vi "FPGA Main.vi"() -> ()   [LabVIEW 2016]
uses:
  Program Files (x86)/National Instruments/LabVIEW 2016/examples/roboRIO/Customized FPGA/Sub VIs/Utilities/Start Boolean.ctl
  <vilib>/Platform/TimedLoop/XDataNode/timing_clust.ctl
  <vilib>/Platform/TimedLoop/XDataNode/nitl_modes.ctl
  <vilib>/Platform/TimedLoop/XDataNode/wakeup.ctl
  <vilib>/rvi/Emulation/niFpgaGetClockAttributes.vi
  <vilib>/rvi/Emulation/niFpgaSctlEmulationGetInTimedLoop.vi
  <vilib>/rvi/Emulation/niFpgaEmulationReportErrorSimple.vi
  <vilib>/rvi/Emulation/niFpgaProcessEmulError.vi
  <vilib>/rvi/Emulation/niFpgaCriticalErrorInLSC.vi
  <vilib>/rvi/eio/common/nirviEmuTemplateMethod_errors.vi
  <vilib>/rvi/Emulation/niFpgaEmulationIsFPGAContextNoSignature.vi
  <vilib>/rvi/errors/niFpgaSetErrorForExecOnDevCompSimple.vi
  <vilib>/rvi/eio/common/nirviEmuReportErrorAndStop.vi
  <vilib>/rvi/DataTransferAndStorage/Container/Common/niFpgaContainerGetUniqueNameForEmu.vi
  <vilib>/rvi/FIFO/Fifo_Resource/nirvififoEmulationSetSize.vi
  <vilib>/rvi/FIFO/Fifo_Resource/nirviFifoEmulationQueueMgr.vi
  <instcachedir>/0/nirviFifoEmulationQueueMgr_E5CAEC123FF24DC58D834DCA3CDAA9B5.lvgen/nirviFifoEmulationQueueMgr_E5CAEC123FF24DC58D834DCA3CDAA9B5_000.vi
  <vilib>/Utility/error.llb/Clear Errors.vi
  <vilib>/rvi/FIFO/Fifo_Resource/nirvififoEmulationCreateLock.vi
  <vilib>/rvi/FIFO/Fifo_Resource/nirvififoEmulationObtainLock.vi
  <vilib>/rvi/FIFO/Fifo_Resource/nirvififoEmulationReleaseLock.vi
  <vilib>/rvi/occurrence/nirviWaitOnOccurrenceBase.vi
  <vilib>/rvi/errors/nirviReportUnexpectedCaseInternalError.vi
  <vilib>/rvi/errors/nirviReportUnexpectedCaseInternalError (U32).vi
  <vilib>/rvi/FIFO/Fifo_Resource/nirvififoEmulationDetermineInputValidOut.vi
  <vilib>/rvi/DataTransferAndStorage/Container/Common/niFpgaContainerExecOnDevCompGetState.vi
  <vilib>/rvi/interface/RandomDataEmulation/niFpgaRandomDataHandleErrors.vi
  <vilib>/rvi/DataTransferAndStorage/Container/Common/niFpgaContainerSetEmuInfo.vi
  <instcachedir>/0/nirviFifoEmulationQueueMgr_E5CAEC123FF24DC58D834DCA3CDAA9B5.lvgen/nirviFifoEmulationQueueMgr_E5CAEC123FF24DC58D834DCA3CDAA9B5_003.vi
  <vilib>/rvi/Memory/Memory_Emulation/niFpgaMemoryEmulationCacheClearOnFirstRun.vi
  <vilib>/rvi/Memory/Memory_Emulation/nirvimemoryEmulationManagerCache_MakeExclusive.vi
  <vilib>/rvi/Memory/Memory_Emulation/niFpgaMemoryEmulationValidateCache.vi
  <vilib>/rvi/Memory/Memory_Emulation/nirvimemoryEmulationManagerCache_InsertValue.vi
  <vilib>/rvi/Memory/Memory_Emulation/nirvimemoryEmulationManagerCache_ReleaseExclusive.vi
  <vilib>/rvi/Memory/Memory_Emulation/nirvimemoryEmulationManagerCache_GetValue.vi
  <vilib>/rvi/Memory/Memory_Emulation/nirvimemoryEmulationManagerCache_SetValue.vi
  <vilib>/eio/EIONode/EIONode.xnode
  <vilib>/rvi/DataTransferAndStorage/Container/XNode/niFpgaContainer.xnode
  <vilib>/rvi/FIFO/Fifo_Resource/nirvififoEmulationRead.vi
  <vilib>/rvi/FIFO/Fifo_Resource/nirvififoEmulationWrite.vi
  <vilib>/rvi/FIFO/Fifo_Resource/niFpgaFifoEmulationRefIn.vi
  <vilib>/rvi/LocalResourceManager/LocalResourceManager.xnode
  <vilib>/rvi/DataTransferAndStorage/Register/Emulation/niFpgaRegisterEmulationRefIn.vi
  <vilib>/Platform/TimedLoop/XDataNode/XDataNode.xnode
  <vilib>/eio/EIOMethodNode/EIOMethodNode.xnode
  <vilib>/Platform/TimedLoop/XDataNode/XDNodeRunTimeDep.lvlib
panel:
  out "ODrive Encoder ready":bool
  in  "SPI.SPI.DATO":u16
  out "SPI.SPI.DATI":u16
  in  "SPI.SPI.CNFG":u16 format="%016b"
  in  "SPI.SPI.CNT":u16
  in  "SPI.SPI.GO":T1
  out "SPI.SPI.STAT":u8 format="%08b"
  in  "DIO.SPI_CS3:0.OUT":u8 format="%08b"
  in  "DIO.SPI_CS3:0.DIR":u8 format="%08b"
  out "DIO.SPI_CS3:0.IN":u8 format="%08b"
  in  "IRQ.TIMER.SETTIME":T1
  in  "IRQ.TIMER.WRITE":u32
  out "IRQ.TIMER.READ":u32
  out "SYS.AI.RDY":bool
  out "SYS.ACC.RDY":bool
  out "SYS.RDY":bool
  in  "MotorsON":bool=TRUE
  in  "ODrive RT Control":bool
  out "Position Axis1":i16
  out "Velocity Axis0":i16
  out "ODrive State":u8
  out "ODrive Error Flags":bool[](array[boolean])
  out "ODrive Errors":u32
  out "IMU_String":u8[](array[numeric])
  out "User Button":bool
  in  "Comm LED Red":bool
  in  "Comm LED Green":bool
  in  "IMU ON?":bool
  out "Read: UWB Char":u8
  out "Read: New UWB Data":bool
  in  "Write: UWB Char":u8
  in  "Write: UWB Data":bool
  out "Current speed":sgl
  out "HallSensorValue":u8
  out "Channel 7 position":u8
  out "Channel 6 position":u8
  out "Channel 5 position":u8
  out "Channel 4 position":u8
  out "Value Channel 0":i32
  in  "Rear wheel motor OFF?":bool=TRUE
  out "Value Channel 2":i32
  out "Value Channel 3":i32
  # "SPI"
  # "System"
  # "FPGA Timer"
  # "SPI CS DIO"
  # "RC"
  # "LEDS and user button"
  # "IMU"
  # "UWB"
  # "LQR"
  # "Steering"
  # "Rear wheel"
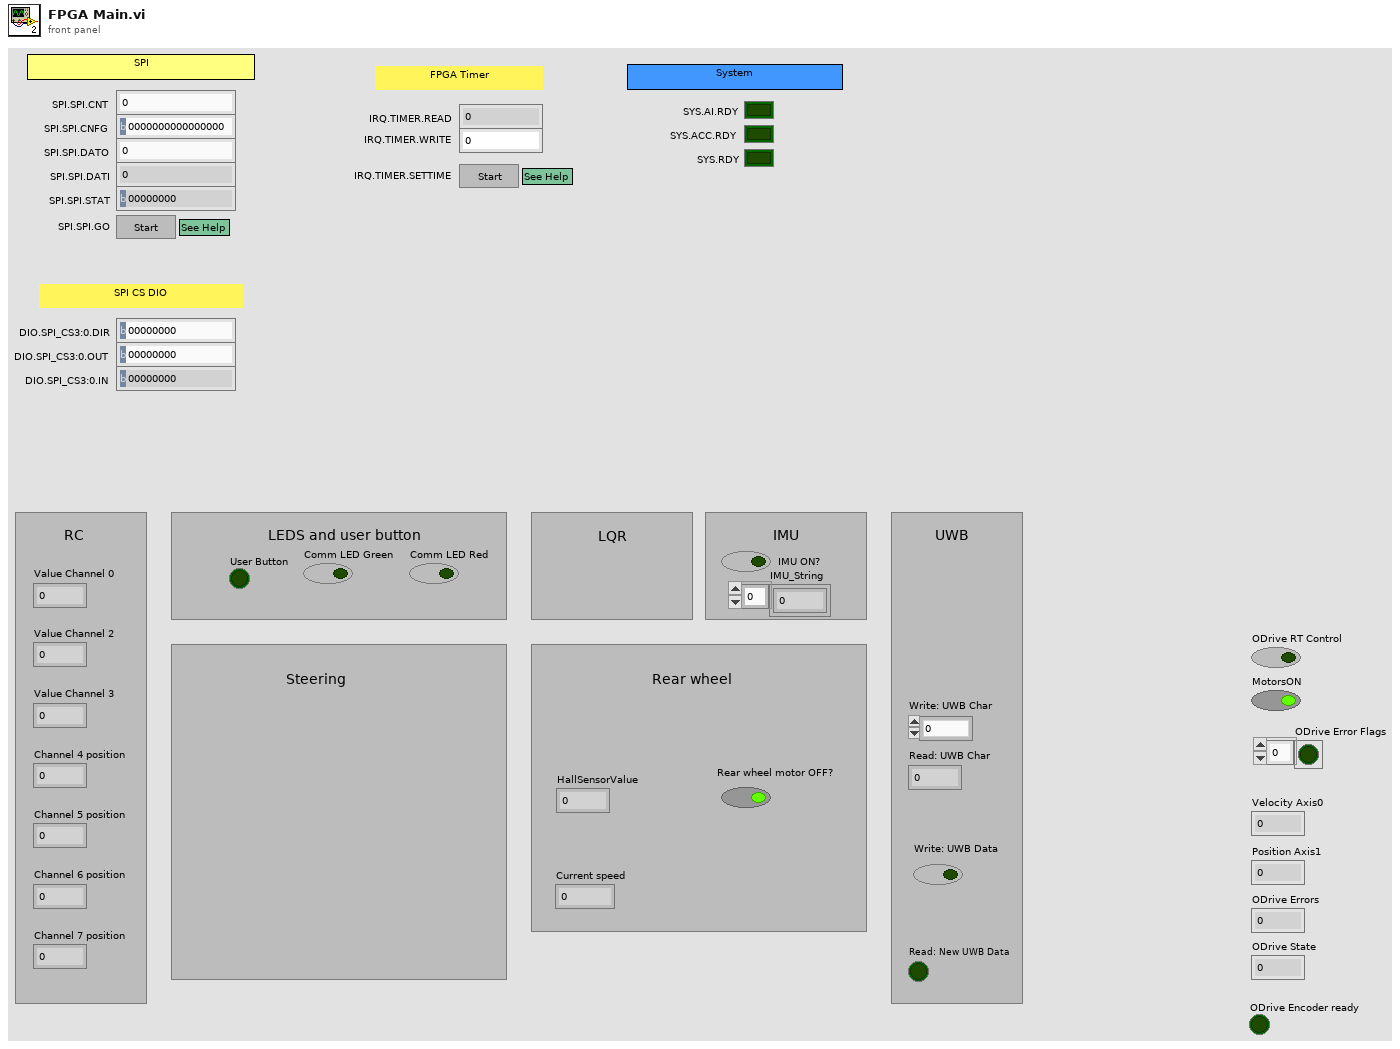
[diagram p1: front panel]
types:
  T1 = typedef "Start Boolean.ctl" = bool
  T2 = typedef "XDNodeRunTimeDep.lvlib/timing_clust.ctl" = cluster{"Expected End [f-1]":u64, "Actual End [f-1]":u64, "Finished Late? [f-1]":bool, "Expected End [i-1]":u64, "Actual End [i-1]":u64, "Finished Late? [i-1]":bool, "Expected Start [i]":u64, "Actual Start [i]":u64, "Expected Start [f]":u64, "Actual Start [f]":u64, "Source Name":string, "Structure Name":string, "Period":i64, "Deadline":i64, "Offset":i64, "Start":i64, "Priority":i32, "Timeout":i32, "Mode":T3, "Wakeup Reason":T4, "Error":errorcluster, "Source Type":string, "Secondary Source Type":string, "Global End Time":u64, "Global Start Time":u64, "Frame Duration":u64, "Iteration Duration":u64, "Assigned CPU":i32, "I/O Scan Engine Mode":u32}
  T3 = typedef "XDNodeRunTimeDep.lvlib/nitl_modes.ctl" = enum32{"No Change", "Process missed periods, maintain original phase", "Discard missed periods, maintain original phase", "Process missed periods, ignore original phase", "Discard missed periods, ignore original phase"}
  T4 = typedef "XDNodeRunTimeDep.lvlib/wakeup.ctl" = enum32{"Normal", "Aborted", "Asynchronous wakeup", "Timing source error", "Timed loop error", "Timeout"}
  T5 = cluster{"ASCII command":u8, "Flags":u8, "Value":i16}
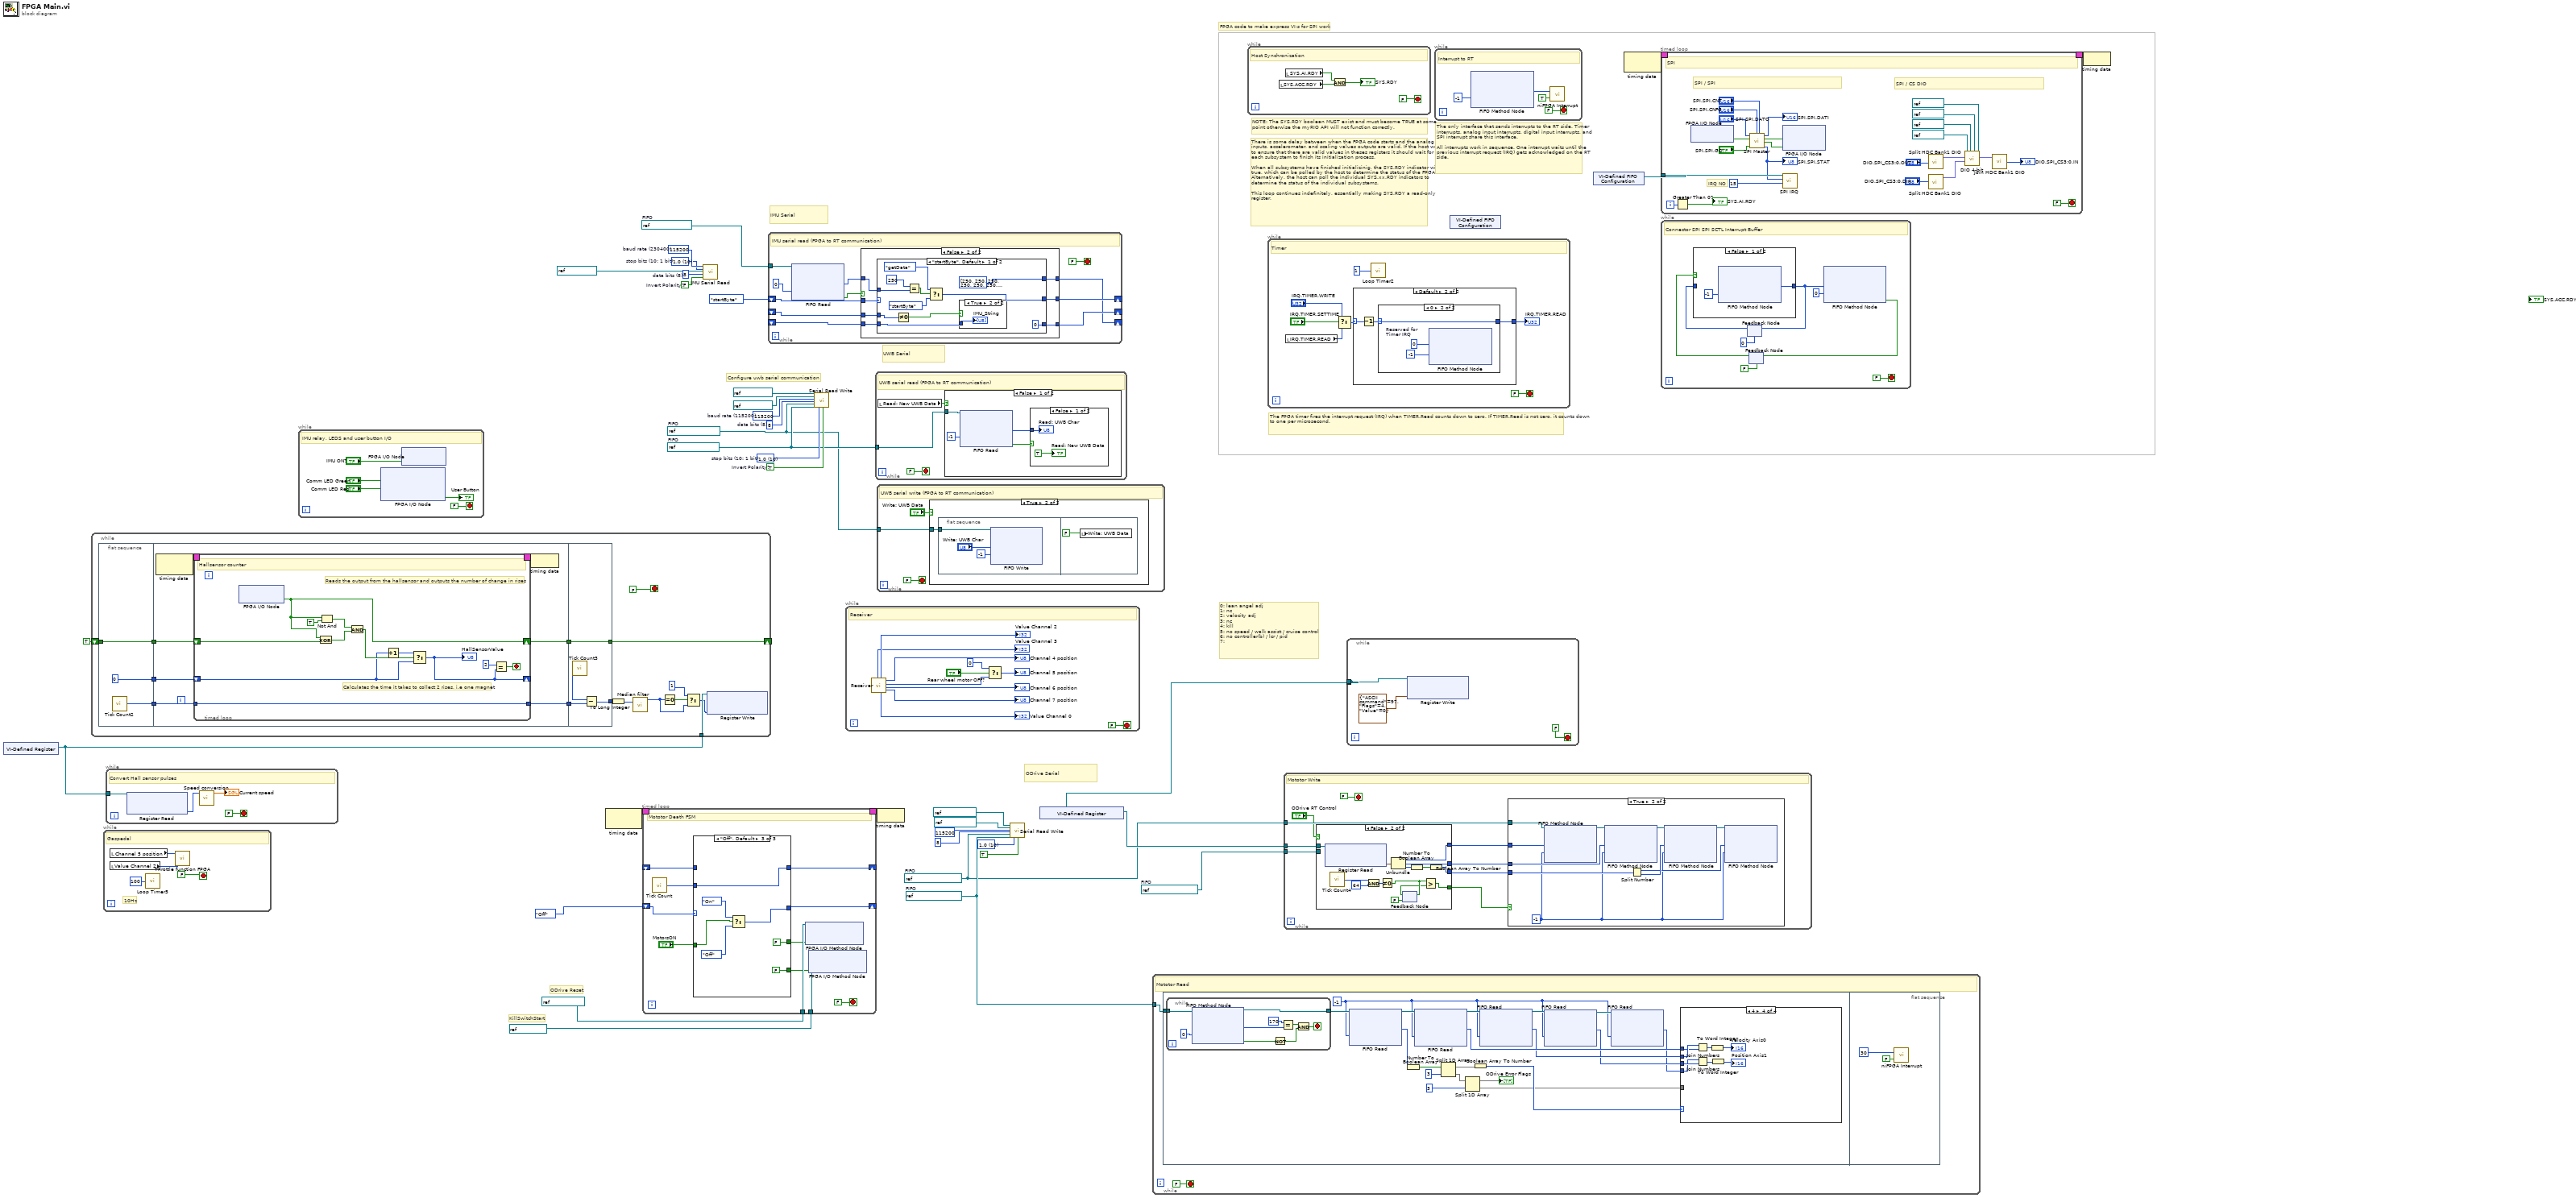
[diagram p0: block diagram]
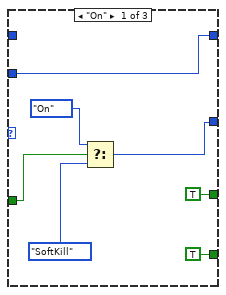
[diagram p5: hidden frame]
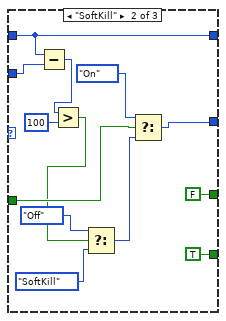
[diagram p6: hidden frame]
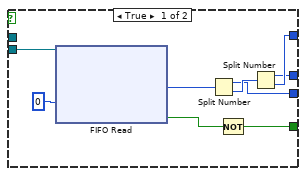
[diagram p8: hidden frame]
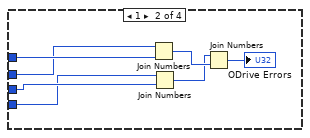
[diagram p10: hidden frame]
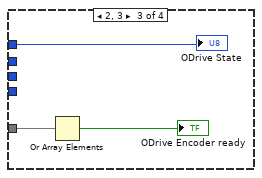
[diagram p11: hidden frame]
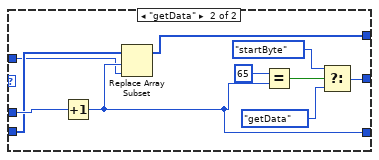
[diagram p14: hidden frame]
diagram:
  w11 = refnum<k21> "RT to ODrive FIFO"  # FIFO
  w16 = u16 10 items=["1.0"=10, "1.5"=15, "2.0"=20] ("stop bits (10: 1 bit)")
  w14 = refnum<k21> "Read FIFO ODrive"  # FIFO
  w12 = refnum<k21> "Write FIFO ODrive"  # FIFO
  w21 = refnum<k21> "Write FIFO UWB"  # FIFO
  w22 = refnum<k21> "Read FIFO UWB"  # FIFO
  w33 = refnum<k21> "Read FIFO IMU"  # FIFO
  w29 = FALSE  # Invert Polarity?
  w30 = 8  # data bits (8)
  w31 = u16 10 items=["1.0"=10, "1.5"=15, "2.0"=20]  # stop bits (10: 1 bit)
  w32 = u32 115200  # baud rate (230400)
  w23 = TRUE  # Invert Polarity?
  w24 = u16 10 items=["1.0"=10, "1.5"=15, "2.0"=20]  # stop bits (10: 1 bit)
  w25 = 8  # data bits (8)
  w26 = u32 115200  # baud rate (115200)
  # "FPGA code to make express VI:s for SPI work"
  # "The FPGA timer fires the interrupt request (IRQ) when TIMER.Read counts down to zero. If TIMER.Read is not zero, it counts down to one per microsecond."
  # "The only interface that sends interrupts to the RT side. Timer interrupts, analog input interrupts, digital input interrupts, and SPI interrupt share this interface.\n\nAll interrupts work in sequence. One interrupt waits until the previous interrupt request (IRQ) gets acknowledged on the RT side."
  # "NOTE: The SYS.RDY boolean MUST exist and must become TRUE at some point otherwise the myRIO API will not function correctly."
  # "There is some delay between when the FPGA code starts and the analog inputs, accelerometer, and scaling values outputs are valid. If the host wants to ensure that there are valid values in theses registers it should wait for each subsystem to finish its initialization process. \n\nWhen all subsystems have finished initializinig, the SYS.RDY indicator will be true, which can be polled by the host to determine the status of the FPGA. Alternatively, the host can poll the individual SYS.xx.RDY indicators to determine the status of the individual subsystems.\n\nThis loop continues indefinitely, essentially making SYS.RDY a read-only register."
  # "0: lean angel adj\n1: nc\n2: velocity adj\n3: nc\n4: kill\n5: no speed / walk assist / cruise control\n6: no controller(b) / lcr / pid\n7:"
  # "KillSwitchStart"
  # "ODrive Reset"
  # "ODrive Serial"
  # "Configure uwb serial communication"
  # "IMU Serial"
  # "UWB Serial"
  n1 = xnode "VI-Defined Register"() -> ("Register Out"=w4:refnum<k21>)
  n2 = while {
    shift-right: [w49] -> _
    shift-left: TRUE ("DIO/DIO3") -> [w50]
    tunnel: w4 -> [w37]
    stop <- FALSE stop-if-true
    n3 = flat-sequence {
      tunnel: w50 -> [w53]
      tunnel: [w53] -> w48
      tunnel: [u8 0] -> w47
      tunnel: [w51] -> w46
      tunnel: w48 -> [w58]
      tunnel: w47 -> [w56]
      tunnel: w46 -> [w55]
      tunnel: [w57] -> w45
      tunnel: [w54] -> w44
      tunnel: [w80] -> w49
      tunnel: w45 -> [w80]
      tunnel: [w79] -> w43
      tunnel: w44 -> [w77]
      frame #0 {
        n4 = call "Tick Count2"() -> ("Tick Count(uSec)"=w51:u32)
      }
      frame #1 {
        n5 = node-c288() -> (w60:T2)  [unwired: 1 in]
        n6 = timed-loop {
          shift-right: [w61] -> _
          shift-left: w56 -> [w62]
          shift-right: [w69] -> w57
          shift-left: w58 -> [w72]
          timing: w60 -> [_]
          timing-out: [_] -> w59
          tunnel: w55 -> [w71]
          tunnel: [w71] -> w54
          stop <- w64 stop-if-true
          # "Calculates the time it takes to collect 2 rises, i.e one magnet"
          # "Reads the output from the hallsensor and outputs the number of change in rises"
          # "Hallsensor counter"
          n7 = xnode "FPGA I/O Node"() -> ("DIO/DIO8"=w69:bool)  [unwired: 1 in, 1 out]
          n8 = Exclusive Or(1:w72, 2:w69) -> (0:w67:bool)
          n9 = Not And(1:TRUE ("y"), 2:w69) -> (0:w68:bool)
          n10 = And(x=w68, y=w67) -> (x .and. y?=w66:bool)
          n11 = Increment(x=w62) -> (x+1=w65:u8)
          n12 = Select(t=w65, s=w66, f=w62) -> (s? t:f=w61:u8)
          "HallSensorValue" <- w61
          n13 = Equal?(x=u8 2, y=w61) -> (x = y?=w64:bool)
        }
        n14 = node-c288(w59) -> ()
      }
      frame #2 {
        n15 = call "Tick Count3"() -> ("Tick Count(uSec)"=w78:u32)
        n16 = Subtract(x=w78, y=w77) -> (x-y=w79:u32)
      }
    }
    n17 = To Long Integer(number=w43) -> (32bit integer=w42:i32)
    n18 = call "Median filter.vi"("Rawdata"=w42) -> ("Filtered element"=w39:i32)  [unwired: 10 in]
    n19 = Equal To 0?(x=w39) -> (x = 0?=w41:bool)
    n20 = Select(t=1, s=w41, f=w39) -> (s? t:f=w36:i32)
    n21 = xnode ("Register Write")("Data"=w36, "Register In"=w37) -> ()  [unwired: 1 out]
  }
  n22 = while {
    stop <- FALSE stop-if-true
    # "10Hz"
    # "Gaspedal"
    n23 = local read "Value Channel 2"() -> (w82:i32)
    n24 = local read "Channel 5 position"() -> (w83:u8)
    n25 = call "Loop Timer5"("Count(mSec)"=u16 100) -> ()  [unwired: 1 out]
    n26 = call "Throttle function FPGA.vi"("RC input"=w82, "Channel 5 position"=w83) -> ()  [unwired: 9 in, 1 out]
  }
  n27 = while {
    tunnel: w4 -> [w86]
    stop <- FALSE stop-if-true
    # "Convert Hall sensor pulses"
    n28 = xnode ("Register Read")("Register In"=w86) -> ("Data"=w85:i32)  [unwired: 1 out]
    n29 = call "Speed conversion.vi"("Filtered data"=w85) -> ("Numeric"=→"Current speed":sgl)  [unwired: 10 in]
  }
  n30 = while {
    stop <- FALSE stop-if-true
    # "IMU relay, LEDS and user button I/O"
    n31 = xnode "FPGA I/O Node"("Comm LED Green"="Comm LED Green", "Comm LED Red"="Comm LED Red") -> ("User Button"=→"User Button":bool)  [unwired: 3 in, 3 out]
    n32 = xnode "FPGA I/O Node"("DIO/DIO3"="IMU ON?") -> ()  [unwired: 1 in, 1 out]
  }
  n33 = node-c288() -> (w10:T2)  [unwired: 1 in]
  n34 = timed-loop {
    timing: w10 -> [_]
    timing-out: [_] -> w9
    shift-right: [w94] -> _
    shift-left: enum16{"On", "SoftKill", "Off"}."Off" -> [w103]
    shift-right: [w102] -> _
    shift-left: _ -> [w100]
    tunnel: refnum<k21> "MXP/DIO13" ("Transmit") -> [w99]
    tunnel: refnum<k21> "DIO/DIO0" ("Transmit") -> [w98]
    stop <- FALSE stop-if-true
    # "Mototor Death FSM"
    n35 = call "Tick Count"() -> ("Tick Count(mSec)"=w101:u16)
    n36 = case shown="\"Off\", Default" w103 {
      tunnel: [w111 w118 w131] -> w102
      tunnel: w101 -> [w111 w119 w131]
      tunnel: w100 -> [_ w118 _]
      tunnel: [TRUE FALSE FALSE] -> w97
      tunnel: [TRUE TRUE FALSE] -> w96
      tunnel: "MotorsON" -> [w108 w122 w128]
      tunnel: [w105 w120 w125] -> w94
      frame "On" {
        n37 = Select(t=enum16{"On", "SoftKill", "Off"}."On", s=w108, f=enum16{"On", "SoftKill", "Off"}."SoftKill") -> (s? t:f=w105:enum16{"On", "SoftKill", "Off"})
      }
      frame "SoftKill" {
        n38 = Subtract(x=w118, y=w119) -> (x-y=w117:u16)
        n39 = Greater?(x=w117, y=u16 100) -> (0:w115:bool)
        n40 = Select(t=enum16{"On", "SoftKill", "Off"}."Off", s=w115, f=enum16{"On", "SoftKill", "Off"}."SoftKill") -> (s? t:f=w112:enum16{"On", "SoftKill", "Off"})
        n41 = Select(t=enum16{"On", "SoftKill", "Off"}."On", s=w122, f=w112) -> (s? t:f=w120:enum16{"On", "SoftKill", "Off"})
      }
      frame "Off", Default {
        n42 = Select(t=enum16{"On", "SoftKill", "Off"}."On", s=w128, f=enum16{"On", "SoftKill", "Off"}."Off") -> (s? t:f=w125:enum16{"On", "SoftKill", "Off"})
      }
    }
    n43 = xnode "FPGA I/O Method Node"("FPGA I/O In"=w99, "Data"=w97) -> ()  [unwired: 1 out]
    n44 = xnode "FPGA I/O Method Node"("FPGA I/O In"=w98, "Data"=w96) -> ()  [unwired: 1 out]
  }
  n45 = call "IMU Serial Read.vi"("baud rate (230400)"=w32, "stop bits (10: 1 bit)"=w31, "Receive"=refnum<k21> "MXP/DIO9", "data bits (8)"=w30, "Invert Polarity?"=w29) -> ()  [unwired: 11 in]
  n46 = while {
    shift-right: [w142] -> _
    shift-left: enum16{"startByte", "getData"}."startByte" -> [w143]
    shift-right: [w138] -> _
    shift-left: _ -> [w139]
    shift-right: [w141] -> _
    shift-left: _ -> [w140]
    tunnel: w33 -> [w137]
    stop <- FALSE stop-if-true
    # "IMU serial read (FPGA to RT communication)"
    n47 = xnode ("FIFO Read")("Timeout"=0, "FIFO In"=w137) -> ("Element"=w135:u8, "Timed Out?"=w134:bool)  [unwired: 1 out]
    n48 = case shown="False" w134 {
      tunnel: w143 -> [w146 w154]
      tunnel: [w146 w153] -> w142
      tunnel: [w145 w152] -> w141
      tunnel: w140 -> [w145 w151]
      tunnel: w139 -> [w147 w150]
      tunnel: [w147 w149] -> w138
      tunnel: w135 -> [_ w148]
      frame True {
      }
      frame False {
        n49 = case shown="\"startByte\", Default" w154 {
          tunnel: w148 -> [w165 w168]
          tunnel: [w161 w175] -> w153
          tunnel: [u8[] [250, 250, 250, 250, 250, 250, 250, 250, 250, 250, 250, 250, 250, 250, 250, 250, 250, 250, 250, 250, 250, 250, 250, 250, 250, 250, 250, 250, 250, 250, 250, 250, 250, 250, 250, 250, 250, 250, 250, 250, 250, 250, 250, 250, 250, 0, 0, 0, 0, 0, 0, 0, 0, 0, 0, 0, 0, 0, 0, 0, 0, 0, 0, 0, 0, 0] ("IMU_String") w167] -> w149
          tunnel: [u8 0 w169] -> w152
          tunnel: w151 -> [w158 w176]
          tunnel: w150 -> [w156 w170]
          frame "startByte", Default {
            n50 = Not Equal To 0?(x=w158) -> (x != 0?=w155:bool)
            n51 = Equal?(x=u8 250, y=w165) -> (x = y?=w157:bool)
            n52 = Select(t=enum16{"startByte", "getData"}."getData", s=w157, f=enum16{"startByte", "getData"}."startByte") -> (s? t:f=w161:enum16{"startByte", "getData"})
            n53 = case shown="True" w155 {
              tunnel: w156 -> [_ w166]
              frame False {
              }
              frame True {
                "IMU_String" <- w166
              }
            }
          }
          frame "getData" {
            n54 = Increment(x=w176) -> (x+1=w169:u8)
            n55 = Replace Array Subset(array=w170, new element=w168, index=w169) -> (w167:u8[])
            n56 = Equal?(x=u8 65, y=w169) -> (x = y?=w173:bool)
            n57 = Select(t=enum16{"startByte", "getData"}."startByte", s=w173, f=enum16{"startByte", "getData"}."getData") -> (s? t:f=w175:enum16{"startByte", "getData"})
          }
        }
      }
    }
  }
  n58 = call "Serial Read Write.vi"("Transmit"=refnum<k21> "MXP/DIO8", "Receive"=refnum<k21> "MXP/DIO7", "baud rate (115200)"=w26, "data bits (8)"=w25, "Transmit FIFO In"=w21, "Receive FIFO In"=w22, "stop bits (10: 1 bit)"=w24, "Invert Polarity?"=w23) -> ()  [unwired: 12 in]
  n59 = while {
    stop <- FALSE stop-if-true
    # "Receiver"
    n60 = call "Receiver.vi"() -> ("Channel 7 position"=→"Channel 7 position":u8, "Channel 6 position"=→"Channel 6 position":u8, "Channel 5 position"=w182:u8, "Channel 4 position"=→"Channel 4 position":u8, "Value Channel 0"=→"Value Channel 0":i32, "Value Channel 2"=→"Value Channel 2":i32, "Value Channel 3"=→"Value Channel 3":i32)  [unwired: 5 in]
    n61 = Select(t=u8 0, s="Rear wheel motor OFF?", f=w182) -> (s? t:f=→"Channel 5 position":u8)
  }
  n62 = while {
    tunnel: w22 -> [w188]
    stop <- FALSE ("Stop UWB") stop-if-true
    # "UWB serial read (FPGA to RT communication)"
    n63 = local read "Read: New UWB Data"() -> (w190:bool)
    n64 = case shown="False" w190 {
      tunnel: w188 -> [w191 _]
      frame False {
        n65 = xnode ("FIFO Read")("Timeout"=-1, "FIFO In"=w191) -> ("Element"=w192:u8, "Timed Out?"=w193:bool)  [unwired: 1 out]
        n66 = case shown="False" w193 {
          tunnel: w192 -> [w196 _]
          frame False {
            "Read: UWB Char" <- w196
            "Read: New UWB Data" <- TRUE ("Read: New Data")
          }
          frame True {
          }
        }
      }
      frame True {
      }
    }
  }
  n67 = while {
    tunnel: w21 -> [w197]
    stop <- FALSE stop-if-true
    # "UWB serial write (FPGA to RT communication)"
    n68 = case shown="True" "Write: UWB Data" {
      tunnel: w197 -> [_ w200]
      frame False {
      }
      frame True {
        n69 = flat-sequence {
          tunnel: w200 -> [w201]
          frame #0 {
            n70 = xnode ("FIFO Write")("Element"="Write: UWB Char", "Timeout"=-1, "FIFO In"=w201) -> ()  [unwired: 2 out]
          }
          frame #1 {
            n71 = local write "Write: UWB Data"(FALSE ("Write: Data Written")) -> ()
          }
        }
      }
    }
  }
  n72 = node-c288(w9) -> ()
  n73 = call "Serial Read Write.vi"("Transmit"=refnum<k21> "MXP/DIO14", "Receive"=refnum<k21> "MXP/DIO15", "baud rate (115200)"=u32 115200, "data bits (8)"=8, "Transmit FIFO In"=w12, "Receive FIFO In"=w14, "stop bits (10: 1 bit)"=w16, "Invert Polarity?"=TRUE) -> ()  [unwired: 12 in]
  n74 = xnode "VI-Defined Register"() -> ("Register Out"=w13:refnum<k21>)
  n75 = while {
    tunnel: w14 -> [w206]
    stop <- FALSE stop-if-true
    # "Mototor Read"
    n76 = flat-sequence {
      tunnel: w206 -> [w213]
      frame #0 {
        w211 = -1 ("Timeout")
        n77 = while {
          tunnel: w213 -> [w246]
          tunnel: [w245] -> w212
          stop <- w247 stop-if-true
          n78 = xnode ("FIFO Method Node")("Timeout"=0, "FIFO In"=w246) -> ("Element"=w251:u8, "Timed Out?"=w252:bool, "FIFO Out"=w245:refnum<k21>)
          n79 = Not(x=w252) -> (.not. x?=w249:bool)
          n80 = Equal?(x=u8 170, y=w251) -> (x = y?=w248:bool)
          n81 = And(x=w248, y=w249) -> (x .and. y?=w247:bool)
        }
        n82 = xnode ("FIFO Read")("Timeout"=w211, "FIFO In"=w212) -> ("Element"=w222:u8, "FIFO Out"=w226:refnum<k21>)  [unwired: 1 out]
        n83 = Number To Boolean Array(number=w222) -> (Boolean array=w218:bool[])
        n84 = xnode ("FIFO Read")("Timeout"=w211, "FIFO In"=w226) -> ("Element"=w217:u8, "FIFO Out"=w225:refnum<k21>)  [unwired: 1 out]
        n85 = Split 1D Array(array=w218, index=3) -> (first subarray=w220:bool[], second subarray=w210:bool[])
        n86 = Split 1D Array(array=w210, index=3) -> (first subarray=→"ODrive Error Flags":bool[], second subarray=w207:bool[])
        n87 = Boolean Array To Number(Boolean array=w220) -> (number=w219:u8)
        n88 = xnode ("FIFO Read")("Timeout"=w211, "FIFO In"=w225) -> ("Element"=w216:u8, "FIFO Out"=w224:refnum<k21>)  [unwired: 1 out]
        n89 = xnode ("FIFO Read")("Timeout"=w211, "FIFO In"=w224) -> ("Element"=w215:u8, "FIFO Out"=w223:refnum<k21>)  [unwired: 1 out]
        n90 = xnode ("FIFO Read")("Timeout"=w211, "FIFO In"=w223) -> ("Element"=w214:u8)  [unwired: 2 out]
        n91 = case shown="4" w219 {
          tunnel: w217 -> [_ w233 w236 w243]
          tunnel: w216 -> [_ w232 _ w244]
          tunnel: w215 -> [_ w231 _ w242]
          tunnel: w214 -> [_ w230 _ w241]
          tunnel: w207 -> [_ _ w235 _]
          frame 0, Default {
          }
          frame 1 {
            n92 = Join Numbers(hi=w232, lo=w233) -> ((hi.lo)=w229:u16)
            n93 = Join Numbers(hi=w230, lo=w231) -> ((hi.lo)=w228:u16)
            n94 = Join Numbers(hi=w228, lo=w229) -> ((hi.lo)=→"ODrive Errors":u32)
          }
          frame 2, 3 {
            n95 = Or Array Elements(Boolean array=w235) -> (logical OR=→"ODrive Encoder ready":bool)
            "ODrive State" <- w236
          }
          frame 4 {
            n96 = Join Numbers(hi=w244, lo=w243) -> ((hi.lo)=w240:u16)
            n97 = Join Numbers(hi=w241, lo=w242) -> ((hi.lo)=w239:u16)
            n98 = To Word Integer(number=w240) -> (16bit integer=→"Velocity Axis0":i16)
            n99 = To Word Integer(number=w239) -> (16bit integer=→"Position Axis1":i16)
          }
        }
      }
      frame #1 {
        n100 = call <vilib>:"niFPGA Interrupt.vi"("Wait Until Cleared (F)"=FALSE, "IRQ Number (0)"=u8 30 ("Element")) -> ()  [unwired: 1 in]
      }
    }
  }
  n101 = while {
    stop <- FALSE stop-if-true
    # "Host Synchronization"
    n102 = local read "SYS.ACC.RDY"() -> (w257:bool)
    n103 = local read "SYS.AI.RDY"() -> (w259:bool)
    n104 = Compound Arithmetic op=AND(w259, w257) -> (→"SYS.RDY":bool)
  }
  n105 = while {
    stop <- FALSE stop-if-true
    # "Timer"
    n106 = local read "IRQ.TIMER.READ"() -> (w263:u32)
    n107 = Select(t="IRQ.TIMER.WRITE", s="IRQ.TIMER.SETTIME", f=w263) -> (s? t:f=w261:u32)
    n108 = case shown="Default" w261 {
      selector: w261 -> [w267 w270]
      tunnel: [w267 w268] -> w260
      frame 0 {
      }
      frame Default {
        n109 = Decrement(x=w270) -> (x-1=w269:u32)
        n110 = case shown="0" w269 {
          selector: w269 -> [w271 w274]
          tunnel: [w271 w274] -> w268
          frame Default {
          }
          frame 0 {
            w273 = u8 0  # Reserved for Timer IRQ
            n111 = xnode ("FIFO Method Node")("Element"=w273, "Timeout"=-1) -> ()  [unwired: 1 in, 2 out]
          }
        }
      }
    }
    "IRQ.TIMER.READ" <- w260
    n112 = call "Loop Timer2"("Count(uSec)"=u8 1 ("Count(mSec)")) -> ()  [unwired: 1 out]
  }
  n113 = while {
    tunnel: w13 -> [w281]
    tunnel: w12 -> [w283]
    tunnel: w11 -> [w279]
    stop <- FALSE stop-if-true
    # "Mototor Write"
    n114 = case shown="False" "ODrive RT Control" {
      tunnel: w281 -> [_ w316]
      tunnel: w279 -> [w301 _]
      tunnel: [w296 w311] -> w276
      tunnel: [w298 w314] -> w278
      tunnel: [w297 w313] -> w277
      tunnel: [w294 w306] -> w275
      frame True {
        n115 = xnode ("FIFO Read")("Timeout"=0, "FIFO In"=w301) -> ("Element"=w300:u32, "Timed Out?"=w295:bool)  [unwired: 1 out]
        n116 = Split Number(x=w300) -> (hi(x)=w296:u16, lo(x)=w299:u16)
        n117 = Not(x=w295) -> (.not. x?=w294:bool)
        n118 = Split Number(x=w299) -> (hi(x)=w297:u8, lo(x)=w298:u8)
      }
      frame False {
        n119 = xnode ("Register Read")("Register In"=w316) -> ("Data"=w315:T5)  [unwired: 1 out]
        n120 = call "Tick Count4"() -> ("Tick Count(mSec)"=w309:u16)
        n121 = And(x=w309, y=u16 64) -> (x .and. y?=w307:u16)
        n122 = Not Equal To 0?(x=w307) -> (x != 0?=w305:bool)
        n123 = Unbundle(w315) -> ("ASCII command"=w314:u8, "Flags"=w313:u8, "Value"=w312:i16)
        n124 = feedback-in #1(w305) -> ()
        n125 = feedback #1(FALSE) -> (w304:bool)
        n126 = Number To Boolean Array(number=w312) -> (Boolean array=w310:bool[])
        n127 = Greater?(x=w305, y=w304) -> (0:w306:bool)
        n128 = Boolean Array To Number(Boolean array=w310) -> (number=w311:u16)
      }
    }
    n129 = case shown="True" w275 {
      tunnel: w283 -> [_ w293]
      tunnel: w278 -> [_ w287]
      tunnel: w277 -> [_ w286]
      tunnel: w276 -> [_ w285]
      frame False {
      }
      frame True {
        w284 = -1 ("Timeout")
        n130 = xnode ("FIFO Method Node")("Element"=w287, "Timeout"=w284, "FIFO In"=w293) -> ("FIFO Out"=w292:refnum<k21>)  [unwired: 1 out]
        n131 = xnode ("FIFO Method Node")("Element"=w286, "Timeout"=w284, "FIFO In"=w292) -> ("FIFO Out"=w291:refnum<k21>)  [unwired: 1 out]
        n132 = Split Number(x=w285) -> (hi(x)=w288:u8, lo(x)=w289:u8)
        n133 = xnode ("FIFO Method Node")("Element"=w289, "Timeout"=w284, "FIFO In"=w291) -> ("FIFO Out"=w290:refnum<k21>)  [unwired: 1 out]
        n134 = xnode ("FIFO Method Node")("Element"=w288, "Timeout"=w284, "FIFO In"=w290) -> ()  [unwired: 2 out]
      }
    }
  }
  n135 = while {
    tunnel: [w318] -> _
    tunnel: w13 -> [w318]
    stop <- FALSE stop-if-true
    n136 = xnode ("Register Write")("Data"=T5 {"ASCII command"=97, "Flags"=4, "Value"=0}, "Register In"=w318) -> ()  [unwired: 1 out]
  }
  n137 = while {
    stop <- FALSE stop-if-true
    # "Interrupt to RT"
    n138 = xnode ("FIFO Method Node")("Timeout"=-1) -> ("Element"=w322:u8)  [unwired: 1 in, 2 out]
    n139 = call <vilib>:"niFPGA Interrupt.vi"("Wait Until Cleared (F)"=TRUE, "IRQ Number (0)"=w322) -> ()  [unwired: 1 in]
  }
  n140 = xnode "VI-Defined FIFO Configuration"() -> ()  [unwired: 1 out]
  n141 = xnode "VI-Defined FIFO Configuration"() -> ("FIFO Out"=w1:refnum<k21>)
  n142 = node-c288() -> (w3:T2)  [unwired: 1 in]
  n143 = timed-loop {
    timing: w3 -> [_]
    timing-out: [_] -> w2
    tunnel: w1 -> [w328]
    i -> [w325]
    stop <- FALSE stop-if-true
    # "IRQ NO"
    # "SPI / CS DIO"
    # "SPI / SPI"
    # "SPI"
    n144 = Greater Than 0?(x=w325) -> (x > 0?=→"SYS.AI.RDY":bool)
    n145 = xnode "FPGA I/O Node"() -> ("SPI MISO"=w345:bool)  [unwired: 1 in, 1 out]
    n146 = call "SPI Master.vi"("Count"="SPI.SPI.CNT", "Configuration"="SPI.SPI.CNFG", "Start?"="SPI.SPI.GO", "MISO"=w345, "Data Out"="SPI.SPI.DATO") -> ("Status"=w326:u8, "SCLK"=w339:bool, "MOSI"=w340:bool, "Data In"=→"SPI.SPI.DATI":u16)  [unwired: 3 in]
    "SPI.SPI.STAT" <- w326
    n147 = xnode "FPGA I/O Node"("SPI MOSI"=w340, "SPI CLK"=w339) -> ()  [unwired: 2 in, 2 out]
    n148 = call "SPI IRQ.vi"("SPI.A.IRQ.NO"=u8 15 ("SPI.SPI.IRQ.NO"), "SPI.STAT"=w326, "FIFO In"=w328) -> ()  [unwired: 9 in]
    n149 = call "Split HDC Bank1 DIO.vi"("IN 7:0"="DIO.SPI_CS3:0.OUT") -> ("OUT 3:0"=w335:fxp<+,4,4>)  [unwired: 2 out]
    n150 = call "Split HDC Bank1 DIO.vi"("IN 7:0"="DIO.SPI_CS3:0.DIR") -> ("OUT 3:0"=w334:fxp<+,4,4>)  [unwired: 2 out]
    n151 = call "DIO 4-bit.vi"("DIO0 Refnum"=refnum<k21> "SPI CS0", "DIO1 Refnum"=refnum<k21> "SPI CS1" ("DIO0 Refnum"), "DIO2 Refnum"=refnum<k21> "SPI CS2" ("DIO0 Refnum"), "DIR 3:0"=w334, "OUT 3:0"=w335, "DIO3 Refnum"=refnum<k21> "SPI CS3" ("DIO0 Refnum")) -> ("IN 3:0"=w333:fxp<+,4,4>)  [unwired: 5 in]
    n152 = call "Join HDC Bank1 DIO.vi"("IN 3:0"=w333) -> ("OUT 7:0"=→"DIO.SPI_CS3:0.IN":u8)  [unwired: 2 in]
  }
  n153 = while {
    stop <- FALSE stop-if-true
    # "Connector SPI SPI SCTL Interrupt Buffer"
    n154 = feedback #2(u8 0 ("Element")) -> (w352:u8)
    n155 = feedback #3(FALSE ("Timed Out?")) -> (w356:bool)
    n156 = case shown="False" w356 {
      tunnel: [w358 w360] -> w353
      tunnel: w352 -> [_ w360]
      frame False {
        n157 = xnode ("FIFO Method Node")("Timeout"=-1) -> ("Element"=w358:u8)  [unwired: 1 in, 2 out]
      }
      frame True {
      }
    }
    n158 = feedback-in #2(w353) -> ()
    n159 = xnode ("FIFO Method Node")("Element"=w353, "Timeout"=0) -> ("Timed Out?"=w354:bool)  [unwired: 1 in, 1 out]
    n160 = feedback-in #3(w354) -> ()
  }
  n161 = node-c288(w2) -> ()
